vi "MathCad_Numeric_Close_Ref.vi"(3 "error in":errorcluster, 5 "Mathcad.INumericValue Reference":refnum<k7>, 6 "IMathcadWorksheet Reference":refnum<k7>) -> (0 "error out":errorcluster, 2 "IMathcadWorksheet Reference":refnum<k7>)   [LabVIEW 2015]
doc: "This closes the reference. Closing references releases that memory space that is being held."
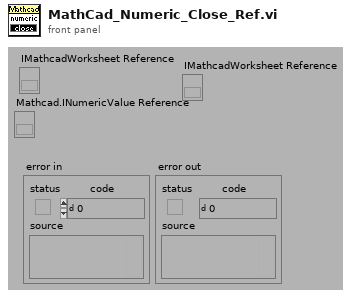
[diagram p1: front panel]
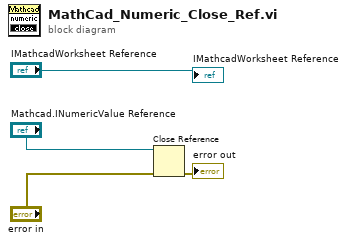
[diagram p0: block diagram]
diagram:
  n1 = Close Reference(reference="Mathcad.INumericValue Reference", error in (no error)="error in") -> (error out=→"error out":errorcluster)
  "IMathcadWorksheet Reference" <- "IMathcadWorksheet Reference"
